vi "Configure GPIB.vi"() -> ()   [LabVIEW 2021]
uses:
  Sub Controls/Instrument.ctl
  Sub Controls/NML GPIB List.ctl
panel:
  in  "Controls":refnum<vi>[](array[refnum])
  in  "GPIB Settings":T3 {"#16"."Parameters" format="%.3e"; "#20"."Parameters" format="%.3e"; "#18"."Parameters" format="%.3e"; "#17"."Parameters" format="%.3e"; "#19"."Parameters" format="%.3e"; "#11"."Parameters" format="%.3e"; "#15"."Parameters" format="%.3e"; "#13"."Parameters" format="%.3e"; "#12"."Parameters" format="%.3e"; "#14"."Parameters" format="%.3e"; "#6"."Parameters" format="%.3e"; "#10"."Parameters" format="%.3e"; "#8"."Parameters" format="%.3e"; "#7"."Parameters" format="%.3e"; "#9"."Parameters" format="%.3e"; "#1"."Parameters" format="%.3e"; "#5"."Parameters" format="%.3e"; "#3"."Parameters" format="%.3e"; "#2"."Parameters" format="%.3e"; "#4"."Parameters" format="%.3e"}
  in  "Done":bool
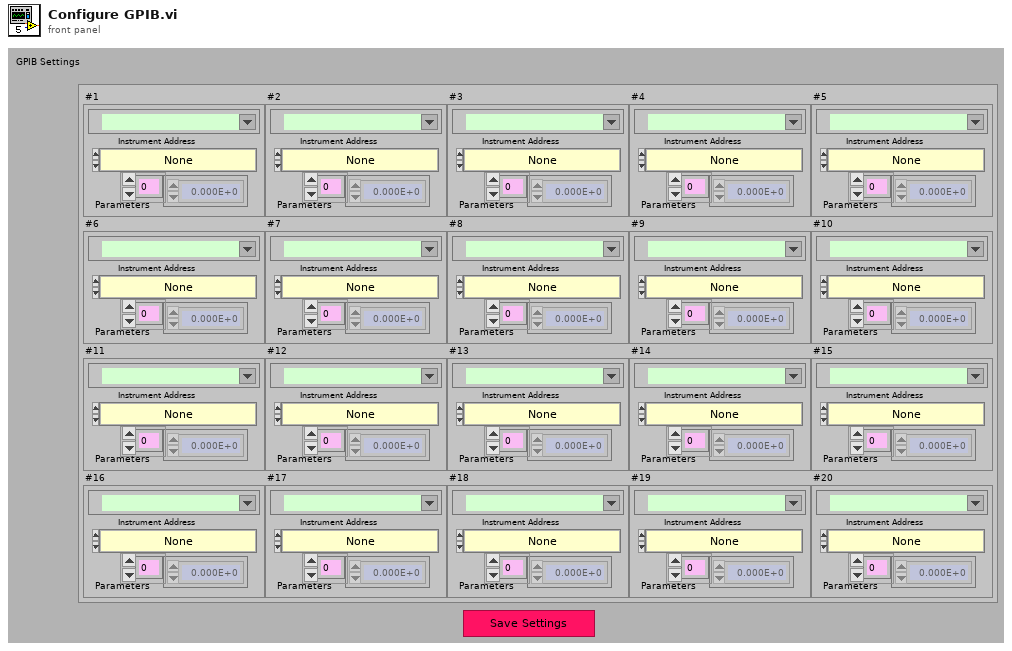
[diagram p1: front panel]
types:
  T1 = typedef "Instrument.ctl" = cluster{"Instrument":T2, "Instrument Address":refnum<visa-resource-name>, "Parameters":dbl[]}
  T2 = typedef "NML GPIB List.ctl" = enum16{"None", "Field", "Field - SCM1", "DMM", "DMM - HP 34401", "Keithley 2XXX", "Running DMM Ave", "Running HP34401", "Running K2XXX Ave", "SRS 830 - CH 1", "SRS 830 - CH1 & 2", "SRS PTC10", "Signal Rec 7265 - X", "Signal Rec 7265 - X&Y", "DRC 93C - Sample", "DRC 93C - Control", "DRC 93C - Sam&Con", "CryoCon Sensor A", "CryoCon Sensor B", "Cond 20C Sensor 1", "Cond 20C Sensor 2", "LS 336 Read", "LS 340 Read", "LS 370 Read", "LS 370 Select", "AVS 46 Bridge", "BLM Rotator Read Position", "Linear Research 700", "LR 700 Select", "Keithley 3330 - LCZ", "A-H Capacitance", "Digital Integrator", "SRS 400 Phot Ctr", "LakeShore VSM", "AMI He Level Meter", "Time Stamp", "Wait", "Invert Current", "K230 Linear V", "K230 VÅB^2", "Temp Ramp", "Power Ramp", "Freq Sweep", "LTC Stable T", "Scanner Step", "IMS Stepper Increment", "BLM Stepper Increment", "Omega CNi32"}
  T3 = cluster{"#1":T1, "#2":T1, "#3":T1, "#4":T1, "#5":T1, "#6":T1, "#7":T1, "#8":T1, "#9":T1, "#10":T1, "#11":T1, "#12":T1, "#13":T1, "#14":T1, "#15":T1, "#16":T1, "#17":T1, "#18":T1, "#19":T1, "#20":T1}
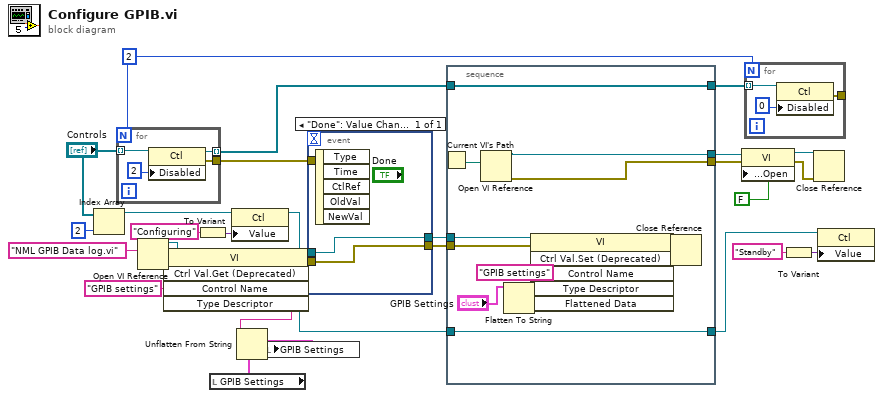
[diagram p0: block diagram]
diagram:
  w11 = 2
  n1 = Index Array(array="Controls", index=2) -> (element=w9:refnum<vi>)
  n2 = for {
    N: w11 -> [_]
    tunnel: "Controls" -> [w33] mode=indexing
    tunnel: [w31] -> w14
    tunnel: [w30] -> w13 mode=indexing
    n3 = property class="Ctl"(reference=w33, "Disabled"=u8 2) -> (reference out=w30:refnum<vi>, error out=w31:errorcluster)  [unwired: 1 in]
  }
  n4 = Open VI Reference(vi path="NML GPIB Data log.vi") -> (vi reference=w27:refnum<vi>, error out=w29:errorcluster)  [unwired: 5 in]
  n5 = invoke class="VI" method="Ctrl Val.Get (Deprecated)"(reference=w27, error in=w29, "Control Name"="GPIB settings") -> (reference out=w2:refnum<vi>, error out=w20:errorcluster, "Get Control Value"=w23:string)  [unwired: 2 in, 2 out]
  n6 = To Variant(anything="Configuring" ("Control Name")) -> (Variant=w7:variant)
  n7 = local read "GPIB Settings"() -> (w24:T3)
  n8 = property class="Ctl"(reference=w9, "Value"=w7) -> (reference out=w1:refnum<vi>)  [unwired: 1 in, 1 out]
  n9 = Unflatten From String(type=w24, binary string=w23) -> (value=w25:T3)  [unwired: 3 in, 2 out]
  n10 = local write "GPIB Settings"(w25) -> ()
  n11 = event shown="[0] \"Done\": Value Change" {
    selector: _ -> [_]
    dyn-events: _ -> [_]
    timeout: _ -> [_]
    tunnel: w2 -> [w35]
    tunnel: [w35] -> w22
    tunnel: [w34] -> w21
    tunnel: w20 -> [w34]
    tunnel: w14 -> [_]
    event "Done": Value Change {
      n12 = event-data() -> ()  [unwired: 1 in, 5 out]
    }
  }
  n13 = stacked-sequence {
    tunnel: w22 -> [w41]
    tunnel: w21 -> [w40]
    tunnel: [w39] -> w17
    tunnel: [w38] -> w15
    tunnel: w13 -> [w37]
    tunnel: [w37] -> w5
    tunnel: [w36] -> w4
    tunnel: w1 -> [w36]
    frame #0 {
      n14 = Current VI's Path() -> (path=w42:path)
      n15 = Open VI Reference(vi path=w42) -> (vi reference=w39:refnum<vi>, error out=w38:errorcluster)  [unwired: 5 in]
      n16 = Flatten To String(anything="GPIB Settings") -> (data string=w46:string, type string=w47:i16[])  [unwired: 3 in, 1 out]
      n17 = invoke class="VI" method="Ctrl Val.Set (Deprecated)"(reference=w41, error in=w40, "Control Name"="GPIB settings", "Type Descriptor"=w47, "Flattened Data"=w46) -> (reference out=w44:refnum<vi>, error out=w43:errorcluster)  [unwired: 1 in, 4 out]
      n18 = Close Reference(reference=w44, error in (no error)=w43) -> ()  [unwired: 1 out]
    }
  }
  n19 = property class="VI"(reference=w17, error in=w15, "Front Panel Window:Open"=FALSE) -> (reference out=w18:refnum<vi>, error out=w19:errorcluster)
  n20 = for {
    N: w11 -> [_]
    tunnel: w5 -> [w51] mode=indexing
    tunnel: [w49] -> _
    n21 = property class="Ctl"(reference=w51, "Disabled"=u8 0) -> (error out=w49:errorcluster)  [unwired: 1 in, 1 out]
  }
  n22 = To Variant(anything="Standby" ("Control Name")) -> (Variant=w3:variant)
  n23 = Close Reference(reference=w18, error in (no error)=w19) -> ()  [unwired: 1 out]
  n24 = property class="Ctl"(reference=w4, "Value"=w3) -> ()  [unwired: 1 in, 2 out]
